vi "Send command Get Port.vi"(8 "error in (no error)":errorcluster, 9 "Puerto":string, 10 "Marca":string, 11 "Serial Device in":refnum<class "Serial Device.lvclass">) -> (0 "error out":errorcluster, 1 "Command":string, 2 "Expected response":string, 3 "Serial Device out":refnum<class "Serial Device.lvclass">)   [LabVIEW 2020, in "Serial Device.lvclass"]
doc: "Se tiene dentro el comando para obtener el estatus del puerto y este sera solo para mandarlo a llamar"
uses:
  Serial Device.lvclass
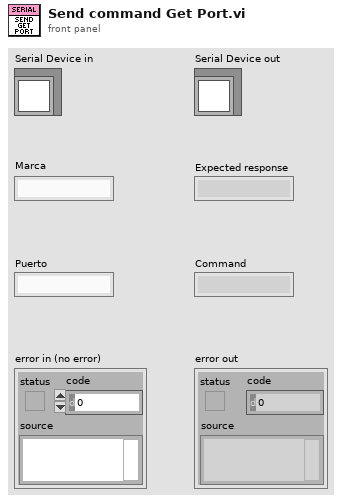
[diagram p1: front panel]
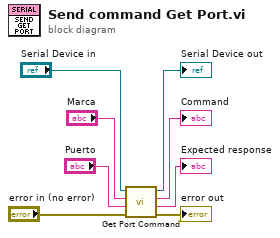
[diagram p0: block diagram]
diagram:
  n1 = call-dynamic "Get Port Command.vi"("error in (no error)"="error in (no error)", "Puerto"="Puerto", "Marca"="Marca", "Serial Device in"="Serial Device in") -> ("error out"=→"error out":errorcluster, "Expected response"=→"Expected response":string, "Command"=→"Command":string, "Serial Device out"=→"Serial Device out":refnum<class "Serial Device.lvclass">)  [unwired: 4 in]
